vi "Set_WheelVelocity.vi"(8 "error in":errorcluster, 10 "fWheelVel":sgl=0.015, 11 "MG17Motor in":refnum<k7>) -> (0 "error out":errorcluster)   [LabVIEW 2014]
doc: "André Romero - 2023\nandretec@ifsc.usp.br\nIFSC - USP"
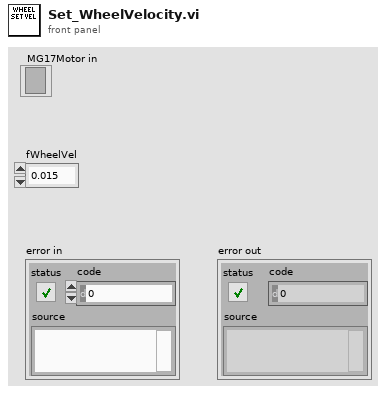
[diagram p1: front panel]
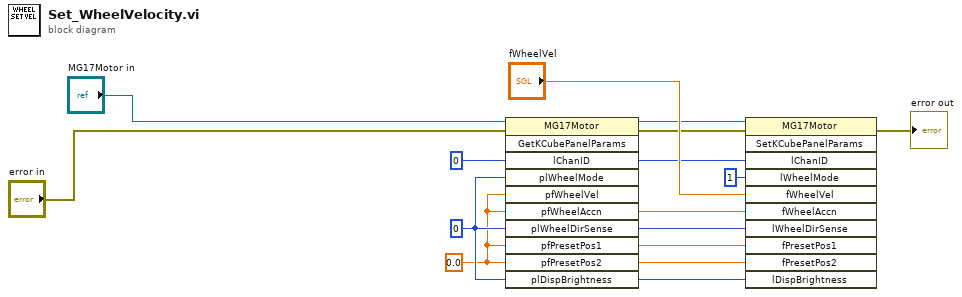
[diagram p0: block diagram]
diagram:
  w2 = 0 ("plWheelMode")
  w1 = sgl 0.0 ("pfPresetPos2")
  n1 = invoke class="MG17Motor" method="GetKCubePanelParams"(reference="MG17Motor in", error in="error in", "lChanID"=0, "plWheelMode"=w2, "pfWheelVel"=w1, "pfWheelAccn"=w1, "plWheelDirSense"=w2, "pfPresetPos1"=w1, "pfPresetPos2"=w1, "plDispBrightness"=w2) -> (reference out=w3:refnum<k7>, error out=w4:errorcluster, "lChanID"=w5:i32, "pfWheelAccn"=w8:sgl, "plWheelDirSense"=w11:i32, "pfPresetPos1"=w10:sgl, "pfPresetPos2"=w9:sgl, "plDispBrightness"=w12:i32)  [unwired: 1 in, 3 out]
  n2 = invoke class="MG17Motor" method="SetKCubePanelParams"(reference=w3, error in=w4, "lChanID"=w5, "lWheelMode"=1, "fWheelVel"="fWheelVel", "fWheelAccn"=w8, "lWheelDirSense"=w11, "fPresetPos1"=w10, "fPresetPos2"=w9, "lDispBrightness"=w12) -> (error out=→"error out":errorcluster)  [unwired: 1 in, 10 out]
